vi "ConvertTestDataToMm.vi"(10 "AScan+Peaks in":cluster{"timebase":dbl[], "data":u16[]}[](array[cluster]), 11 "Value":dbl) -> (3 "Array":cluster{"timebase":dbl[], "data":u16[]}[](array[cluster]))   [LabVIEW 2026]
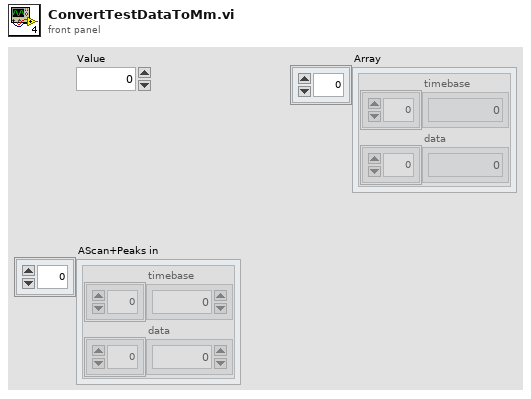
[diagram p1: front panel]
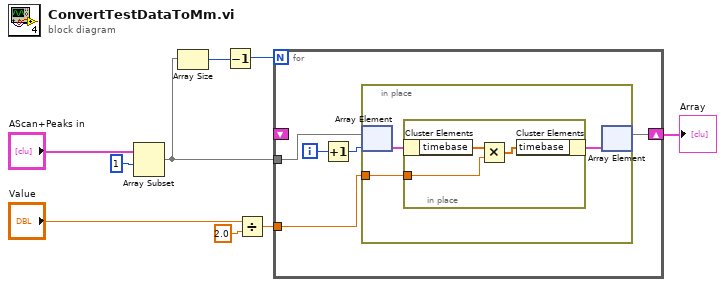
[diagram p0: block diagram]
diagram:
  n1 = Array Subset(array="AScan+Peaks in", index=1) -> (w7:cluster{"timebase":dbl[], "data":u16[]}[])  [unwired: 1 in]
  n2 = Array Size(array=w7) -> (size(s)=w8:i32)
  n3 = Decrement(x=w8) -> (x-1=w1:i32)
  n4 = Divide(x="Value", y=2.0) -> (x/y=w3:dbl)
  n5 = for {
    N: w1 -> [_]
    tunnel: w7 -> [w14]
    tunnel: w3 -> [w13]
    shift-right: [w12] -> w2
    shift-left: _ -> [_]
    i -> [w11]
    n6 = Increment(x=w11) -> (x+1=w10:i32)
    n7 = in-place {
      in-place-border: w13 -> [w16]
      n8 = in-place-array #1(w14, w10) -> (w17:cluster{"timebase":dbl[], "data":u16[]})
      n9 = in-place {
        in-place-border: w16 -> [w19]
        n10 = in-place-cluster #2(w17) -> ("timebase"=w20:dbl[])
        n11 = Multiply(x=w20, y=w19) -> (x*y=w18:dbl[])
        n12 = in-place-cluster #2("timebase"=w18) -> (w15:cluster{"timebase":dbl[], "data":u16[]})
      }
      n13 = in-place-array #1(w15) -> (w12:cluster{"timebase":dbl[], "data":u16[]}[])  [unwired: 1 out]
    }
  }
  "Array" <- w2
